vi "4155C Config SamplingI Measurements.vi"(1 "Standby":T1, 4 "Sample time":dbl min=0.0 max=100000000000.0 format="%.2f", 5 "Display on/off":bool, 6 "Timings":T2={"integration time"=0, "Short/Long integration time"=0.00064, "hold time (sec)"=0.0, "delay time (sec)"=0.0, "Step Time (0 disables)"=0.0, "sweep method"=0, "Pulse period"=0.005, "Base voltage"=0.0, "Pulse width"=0.0005} {"Pulse width" min=0.0005 max=0.1 step=0.0001 format="%.4f"; "Base voltage" min=-100.0 max=100.0 format="%^.4e"; "Pulse period" min=0.005 max=1.0 step=0.0001 format="%.4f"; "sweep method" items=["Continuous", "Pulsed"]; "Step Time (0 disables)" format="%.2f"; "delay time (sec)" min=0.0 format="%.4f"; "hold time (sec)" min=0.0 format="%.4f"; "Short/Long integration time" min=0.0 format="%^.0e"; "integration time" scale=0.0..2.0}, 7 "Num Points":i16=1 min=1 max=1001, 8 "error in (no error)":errorcluster, 9 "Sampling interval":dbl min=0.0 max=100000000000.0 format="%.6f", 11 "VISA session":refnum<visa-resource-name>) -> (0 "error out":errorcluster, 3 "dup VISA resource name":refnum<visa-resource-name>)   [LabVIEW 2016]
doc: "This VI configures the primary sweep source (VAR1) for a sweep mode measurement. \n* This VI does not perform error checking on MEASUREMENT MODE or UNIT TYPE of VAR1, therefore it is the application programmer's responsibility to make certain this VI is used in the proper mode."
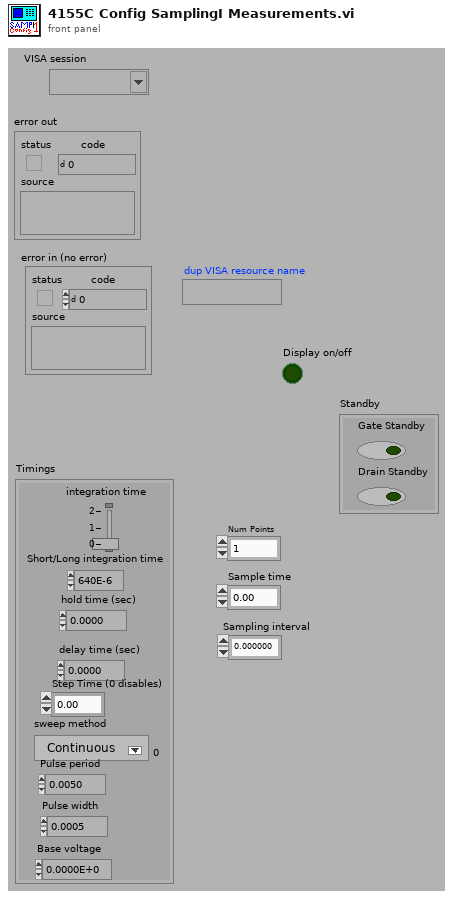
[diagram p1: front panel]
types:
  T1 = cluster{"Gate Standby":bool, "Drain Standby":bool}
  T2 = cluster{"integration time":u32, "Short/Long integration time":dbl, "hold time (sec)":dbl, "delay time (sec)":dbl, "Step Time (0 disables)":dbl, "sweep method":u16, "Pulse period":dbl, "Base voltage":dbl, "Pulse width":dbl}
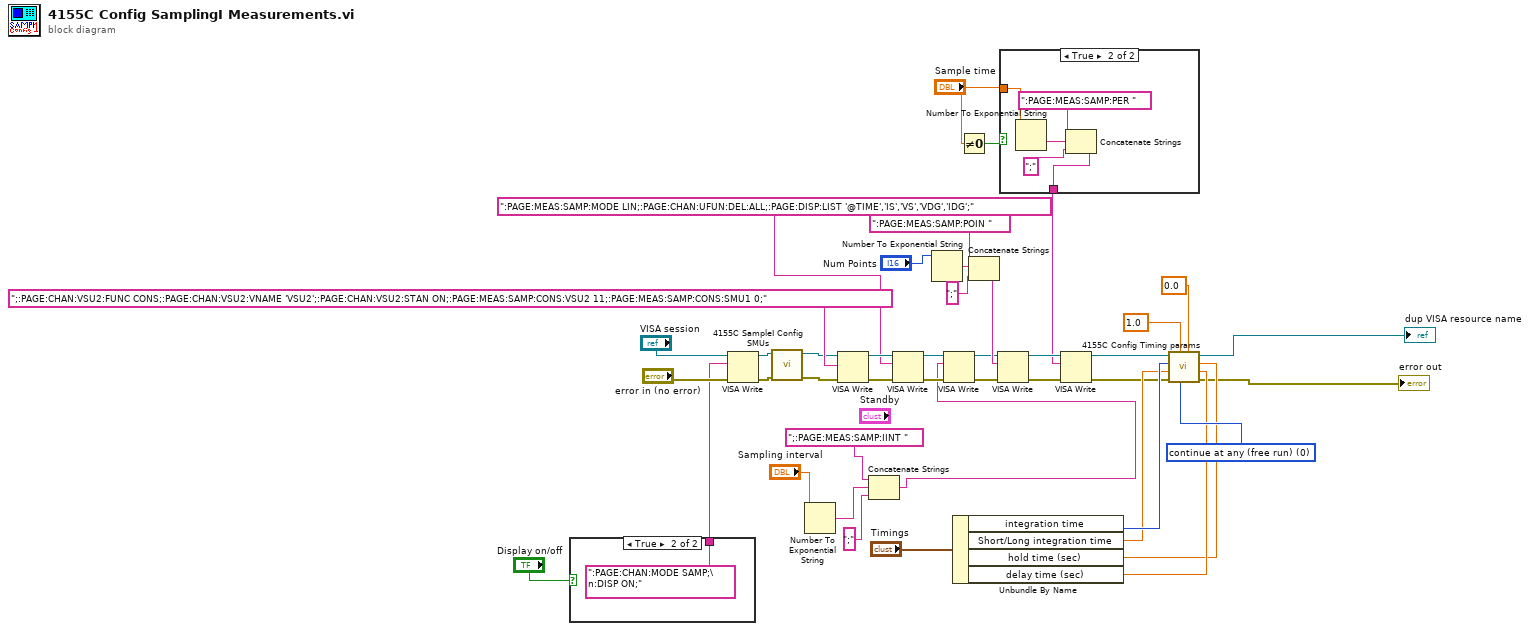
[diagram p0: block diagram]
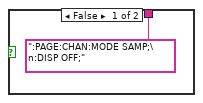
[diagram p2: hidden frame]
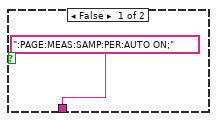
[diagram p3: hidden frame]
diagram:
  w40 = u8 0 items=["continue at any (free run)", "stop at any abnorm", "stop at compliance"] ("stop condition (free run:0)")
  n1 = case shown="True" "Display on/off" {
    tunnel: [":PAGE:CHAN:MODE SAMP;\n:DISP OFF;" ("write buffer (\"\")") ":PAGE:CHAN:MODE SAMP;\n:DISP ON;" ("write buffer (\"\")")] -> w11
    frame False {
    }
    frame True {
    }
  }
  n2 = VISA Write(VISA resource name="VISA session", write buffer=w11, error in (no error)="error in (no error)") -> (VISA resource name out=w29:refnum<visa-resource-name>, error out=w28:errorcluster)  [unwired: 1 out]
  n3 = call "4155C SampleI Config SMUs.vi"("error in (no error)"=w28, "VISA resource name in"=w29) -> ("error out"=w27:errorcluster, "VISA Resource Name out"=w26:refnum<visa-resource-name>)  [unwired: 4 in]
  n4 = Number To Exponential String(number="Sampling interval") -> (E-format string=w10:string)  [unwired: 3 in]
  n5 = VISA Write(VISA resource name=w26, write buffer=";:PAGE:CHAN:VSU2:FUNC CONS;:PAGE:CHAN:VSU2:VNAME 'VSU2';:PAGE:CHAN:VSU2:STAN ON;:PAGE:MEAS:SAMP:CONS:VSU2 11;:PAGE:MEAS:SAMP:CONS:SMU1 0;" ("write buffer (\"\")"), error in (no error)=w27) -> (VISA resource name out=w43:refnum<visa-resource-name>, error out=w42:errorcluster)  [unwired: 1 out]
  n6 = Concatenate Strings(";:PAGE:MEAS:SAMP:IINT ", w10, ";" ("Substring")) -> (w3:string)
  n7 = VISA Write(VISA resource name=w43, write buffer=":PAGE:MEAS:SAMP:MODE LIN;:PAGE:CHAN:UFUN:DEL:ALL;:PAGE:DISP:LIST '@TIME','IS','VS','VDG','IDG';", error in (no error)=w42) -> (VISA resource name out=w2:refnum<visa-resource-name>, error out=w6:errorcluster)  [unwired: 1 out]
  n8 = Number To Exponential String(number="Num Points") -> (E-format string=w24:string)  [unwired: 3 in]
  n9 = VISA Write(VISA resource name=w2, write buffer=w3, error in (no error)=w6) -> (VISA resource name out=w4:refnum<visa-resource-name>, error out=w5:errorcluster)  [unwired: 1 out]
  n10 = Unbundle By Name("Timings") -> ("integration time"=w37:u32, "Short/Long integration time"=w32:dbl, "hold time (sec)"=w38:dbl, "delay time (sec)"=w39:dbl)
  n11 = Not Equal To 0?(x="Sample time") -> (x != 0?=w18:bool)
  n12 = Concatenate Strings(":PAGE:MEAS:SAMP:POIN " ("write buffer (\"\")"), w24, ";" ("Substring")) -> (w20:string)
  n13 = VISA Write(VISA resource name=w4, write buffer=w20, error in (no error)=w5) -> (VISA resource name out=w17:refnum<visa-resource-name>, error out=w16:errorcluster)  [unwired: 1 out]
  n14 = case shown="True" w18 {
    tunnel: "Sample time" -> [_ w50]
    tunnel: [":PAGE:MEAS:SAMP:PER:AUTO ON;" w47] -> w13
    frame False {
    }
    frame True {
      n15 = Number To Exponential String(number=w50) -> (E-format string=w51:string)  [unwired: 3 in]
      n16 = Concatenate Strings(":PAGE:MEAS:SAMP:PER " ("Substring"), w51, ";" ("Substring")) -> (w47:string)
    }
  }
  n17 = VISA Write(VISA resource name=w17, write buffer=w13, error in (no error)=w16) -> (VISA resource name out=w14:refnum<visa-resource-name>, error out=w15:errorcluster)  [unwired: 1 out]
  n18 = call "4155C Config Timing params.vi"("delay time (sec)"=w39, "hold time (sec)"=w38, "Step Time (0 disables)"=0.0, "stop condition (free run:0)"=w40, "wait time parameter"=1.0, "error in (no error)"=w15, "Short/Long integration time"=w32, "integration time"=w37, "VISA session"=w14) -> ("error out"=→"error out":errorcluster, "dup VISA resource name"=→"dup VISA resource name":refnum<visa-resource-name>)  [unwired: 1 in]
